vi "Bridge Bias Set.vi"(8 "error in":errorcluster, 9 "channel index (0: first)":i32, 10 "bias [V]":dbl, 11 "bridge in":T1 {"TWM"."f-list [Hz]" format="%#_6p"}) -> (0 "error out":errorcluster, 3 "bridge out":T1 {"TWM"."f-list [Hz]" format="%#_6p"})   [LabVIEW 2013]
doc: "Set DC bias voltage of selected bias compensator channel."
uses:
  Bridge Session.ctl
  Bridge Type.ctl
  drivers/TWM client/TWM Session.ctl
  drivers/TWM client/TWM parameters.ctl
  drivers/TWM client/Meas Proc QWTB Uncertainty Mode.ctl
  Bridge Bias Session.ctl
  Bridge Bias Type.ctl
  <vilib>/Utility/error.llb/Error Cluster From Error Code.vi
  <vilib>/ErrorRing/Error Ring.xnode
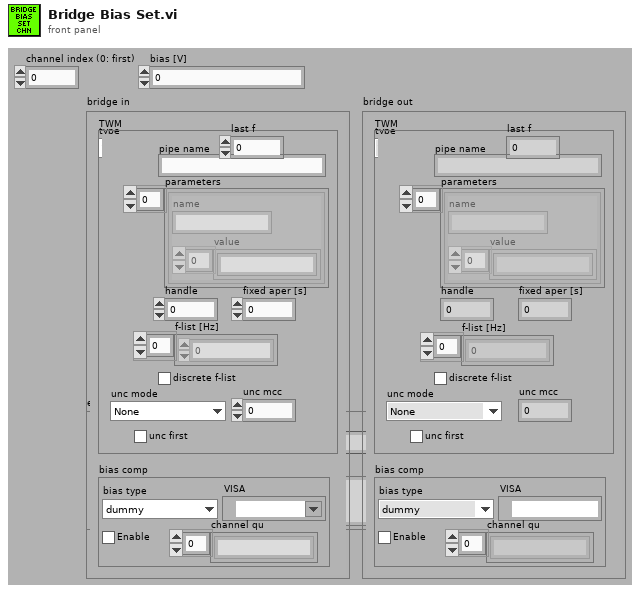
[diagram p1: front panel]
types:
  T1 = typedef "Bridge Session.ctl" = cluster{"type":T2, "TWM":T3, "last f":dbl, "bias comp":T6}
  T2 = typedef "Bridge Type.ctl" = enum16{"TWM client", "dummy"}
  T3 = typedef "TWM Session.ctl" = cluster{"pipe name":string, "parameters":T4[], "handle":i32, "fixed aper [s]":dbl, "f-list [Hz]":dbl[], "discrete f-list":bool, "unc mode":T5, "unc mcc":i32, "unc first":bool}
  T4 = typedef "TWM parameters.ctl" = cluster{"name":string, "value":string[]}
  T5 = typedef "Meas Proc QWTB Uncertainty Mode.ctl" = enum16{"None", "GUF", "Monte Carlo"}
  T6 = typedef "Bridge Bias Session.ctl" = cluster{"bias type":T7, "VISA":refnum<visa-resource-name>, "Enable":bool, "channel qu":string[]}
  T7 = typedef "Bridge Bias Type.ctl" = enum16{"dummy", "CMI LiBbias V1.0"}
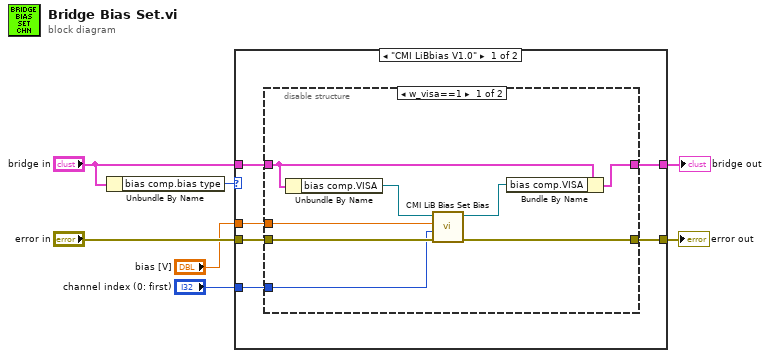
[diagram p0: block diagram]
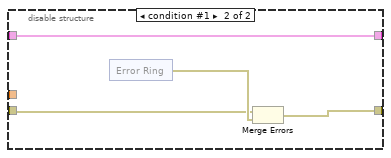
[diagram p2: hidden frame]
diagram:
  n1 = Unbundle By Name("bridge in") -> ("bias comp.bias type"=w7:T7)
  n2 = case shown="\"CMI LiBbias V1.0\"" w7 {
    tunnel: "error in" -> [w11 w32]
    tunnel: [w10 w32] -> w5
    tunnel: "bridge in" -> [w13 w31]
    tunnel: [w12 w31] -> w3
    tunnel: "channel index (0: first)" -> [w9 _]
    tunnel: "bias [V]" -> [w8 _]
    frame "CMI LiBbias V1.0" {
      n3 = disable-structure shown="w_visa==1" {
        disable-tunnel: w13 -> [w21 w22]
        disable-tunnel: [w20 w22] -> w12
        disable-tunnel: w11 -> [w19 w24]
        disable-tunnel: [w18 w23] -> w10
        disable-tunnel: w9 -> [w15 _]
        disable-tunnel: w8 -> [w14 _]
        frame condition #0 (active) {
          n4 = Unbundle By Name(w21) -> ("bias comp.VISA"=w17:refnum<visa-resource-name>)
          n5 = call "CMI LiB Bias Set Bias.vi"("error in"=w19, "channel index (0: first)"=w15, "bias [V]"=w14, "VISA in"=w17) -> ("error out"=w18:errorcluster, "VISA out"=w16:refnum<visa-resource-name>)  [unwired: 6 in]
          n6 = Bundle By Name(cluster=w21, "bias comp.VISA"=w16) -> (w20:T1)
        }
        frame condition #1 {
          n7 = xnode "Error Ring"() -> ("error out"=w25:errorcluster)
          n8 = Merge Errors(w24, w25) -> (w23:errorcluster)
        }
      }
    }
    frame Default {
    }
  }
  "error out" <- w5
  "bridge out" <- w3
